vi "dialog.vi"(4 "Sequence Context":refnum<k7>) -> (0 "error out":errorcluster)   [LabVIEW 2011]
doc: "This VI is an example of a dialog box that is modal to the TestStand main application window using the TestStand Utility VIs. A modal dialog prevents the user from interacting with the TestStand Application until the modal dialog is dismissed."
uses:
  <vilib>/addons/TestStand/_TSUtility.llb/TestStand - Start Modal Dialog (Sequence Context).vi
  <vilib>/addons/TestStand/_TSUtility.llb/TestStand - End Modal Dialog (Sequence Context).vi
panel:
  in  "OK":bool
  # "This VI is an example of a dialog box that is made modal to the TestStand main application window using the TestStand Utility VIs.  A modal dialog prevents the user from interacting with the TestStand application until the dialog is dismissed."
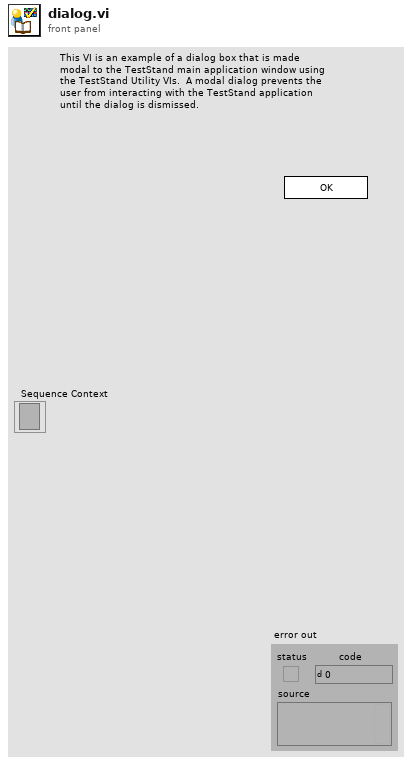
[diagram p1: front panel]
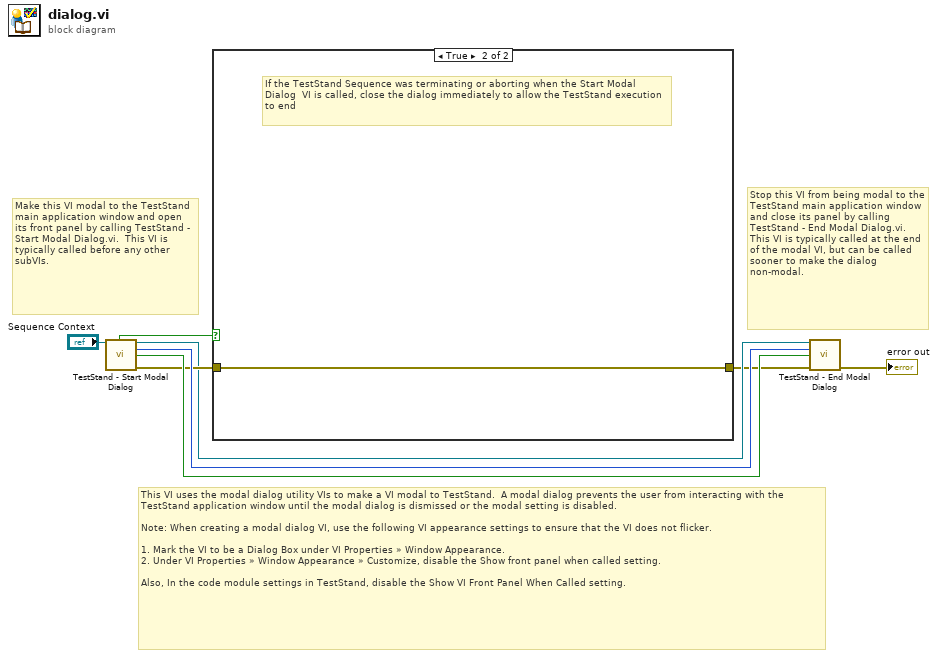
[diagram p0: block diagram]
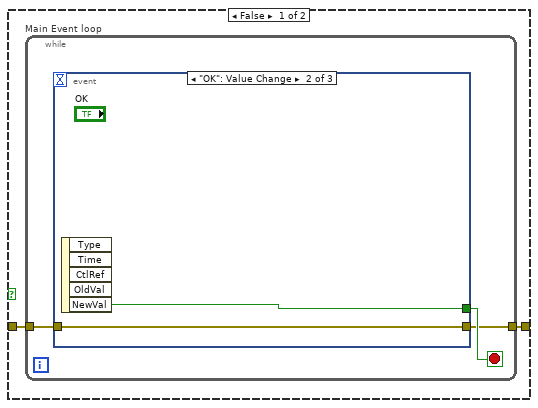
[diagram p2: hidden frame]
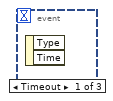
[diagram p3: hidden frame]
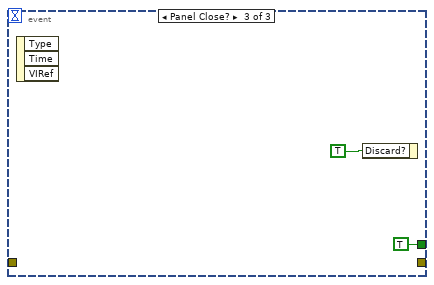
[diagram p4: hidden frame]
diagram:
  # "Make this VI modal to the TestStand main application window and open its front panel by calling TestStand - Start Modal Dialog.vi.  This VI is typically called before any other subVIs."
  # "Stop this VI from being modal to the TestStand main application window and close its panel by calling TestStand - End Modal Dialog.vi.  This VI is typically called at the end of the modal VI, but can be called sooner to make the dialog non-modal."
  # "This VI uses the modal dialog utility VIs to make a VI modal to TestStand.  A modal dialog prevents the user from interacting with the TestStand application window until the modal dialog is dismissed or the modal setting is disabled.\n\nNote: When creating a modal dialog VI, use the following VI appearance settings to ensure that the VI does not flicker.\n\n1. Mark the VI to be a Dialog Box under VI Properties » Window Appearance.\n2. Under VI Properties » Window Appearance » Customize, disable the Show front panel when called setting.\n\nAlso, In the code module settings in TestStand, disable the Show VI Front Panel When Called setting."
  n1 = call-poly <vilib>:"TestStand - Start Modal Dialog.vi"("Sequence Context In"="Sequence Context") -> ("Sequence Context Out"=w2:refnum<k7>, "Modal ID"=w6:i32, "VI Originally Open"=w5:bool, "Should Abort"=w7:bool, "error out"=w4:errorcluster)  [unwired: 2 in, 8 out]
  n2 = case shown="True" w7 {
    tunnel: w4 -> [w10 w18]
    tunnel: [w9 w18] -> w1
    frame False {
      n3 = while "Main Event loop" {
        tunnel: w10 -> [w11]
        tunnel: [w12] -> w9
        stop <- w13 stop-if-true
        n4 = event shown="[1] \"OK\": Value Change" {
          selector: _ -> [_ _ _]
          dyn-events: _ -> [_ _ _]
          timeout: _ -> [_ _ _]
          tunnel: [_ w15 TRUE ("NewVal")] -> w13
          tunnel: [_ w14 _] -> w12
          tunnel: w11 -> [_ w14 _]
          event Timeout {
            n5 = event-data() -> ()  [unwired: 1 in, 2 out]
          }
          event "OK": Value Change {
            n6 = event-data() -> ("NewVal"=w15:bool)  [unwired: 1 in, 4 out]
          }
          event Panel Close? {
            n7 = event-data() -> ()  [unwired: 1 in, 3 out]
            n8 = event-data("Discard?"=TRUE ("NewVal")) -> ()  [unwired: 1 in, 1 out]
          }
        }
      }
    }
    frame True {
      # "If the TestStand Sequence was terminating or aborting when the Start Modal Dialog  VI is called, close the dialog immediately to allow the TestStand execution to end"
    }
  }
  n9 = call-poly <vilib>:"TestStand - End Modal Dialog.vi"("Sequence Context In"=w2, "Modal ID"=w6, "VI Originally Open"=w5, "error in (no error)"=w1) -> ("error out"=→"error out":errorcluster)  [unwired: 1 in, 10 out]
